vi "querey source settings menu.vi"(0 "Enable":bool=TRUE, 1 "subvi?":bool, 2 "Old Settings":T1, 5 "error in (no error)":errorcluster) -> (14 "Output cluster":T4={"Integer Timestamp"=0, "Einzel Voltage"=0.0, "Needle Voltage"=0.0, "Frequency"=1.0, "Width (ms) : 0.1 "=0.05, "Desired Amplitude (V)"=0.0, "X Voltage"=0.0, "Y Voltage"=0.0, "Settings ID"="", "ID#"=0} {"Needle Voltage" min=0.0 max=10.0 step=0.01 format="%.2g"; "Y Voltage" min=0.0 max=9.0 step=0.01 format="%.2g"; "X Voltage" min=0.0 max=9.0 step=0.01 format="%.2g"; "Einzel Voltage" min=0.0 max=10.0 step=0.01 format="%.2g"; "Desired Amplitude (V)" min=0.0 max=10.0 step=0.01 format="%5.2f"; "Width (ms) : 0.1" min=0.05 max=5.0 step=0.01 format="%6.2f"; "Frequency" min=1.0 max=100.0 step=0.01 format="%.1f"}, 15 "Cancel loading":bool caption="Cancel", 18 "OK":bool, 19 "error out":errorcluster)   [LabVIEW 2013]
doc: "Displays a standard dialog box that prompts users to enter information, such as a user name and password.\n--------------------\n\nThis Express VI is configured as follows:\n\nMessage to Display to the User:\nThe inputs are: \nNumber: Upper Timestamp Range\nNumber: Lower Timestamp Range\nNumber: Settings ID"
uses:
  Controls/dust_soruce_control.ctl
  <vilib>/Utility/miscctls.llb/LVPointTypeDef.ctl
  <vilib>/addons/database/Auxilliary.llb/DB Tools Cursor Type.ctl
  <vilib>/addons/database/Connection.llb/Conn Execute.vi
  <vilib>/addons/database/Recordset.llb/Rec Fetch Recordset Data (R).vi
  <vilib>/addons/database/Recordset.llb/Rec Destroy - Connection.vi
  <vilib>/addons/database/_DB Variant To Data/Database Variant To Data.xnode
  <vilib>/regexp/Match Regular Expression.xnode
  <vilib>/addons/database/NI_Database_API.lvlib
panel:
  out "Small Settings":cluster{"String":string, "Value":dbl}[](array[cluster])
  in  "Clear Filter":bool
  in  "Tag Filter":T2
  in  "Settings ID Type":T3(radio)
  in  "OK2":bool
  in  "Cancel":bool
  in  "Settings ID":i32(ring) items=["Any Settings ID."=-1, "Big Accelerator:  (time: 6/12/2014 3:08:20 PM; DT: Graphite-2-1)"=11, "Big Accelerator: test (time: 6/12/2014 11:46:17 AM;DT: Graphite-2-1)"=10, "Big Accelerator: test (time: 6/12/2014 10:56:33 AM;DT: Graphite-2-1)"=8, "Big Accelerator:  (time: 6/12/2014 10:56:28 AM;DT: Graphite-2-1)"=7, "Big Accelerator: olivine (saved at  1/29/2014 1:59:55 PM)"=6, "Big Accelerator: olivine (saved at  1/29/2014 1:53:03 PM)"=4, "Big Accelerator: test (saved at  1/29/2014 1:49:28 PM)"=2]
  in  "Lower Timestamp Range":timestamp
  in  "Upper Timestamp Range":timestamp
  out "Settings":cluster{"String":string, "Value":dbl}[](array[cluster])
  in  "Einzel Voltage":dbl
  in  "Needle Voltage":dbl
  in  "Frequency":dbl
  in  "Width (ms) : 0.1":dbl
  in  "Desired Amplitude (V)":dbl
  in  "X Voltage":dbl
  in  "Y Voltage":dbl
  out "Settings to be loaded":string
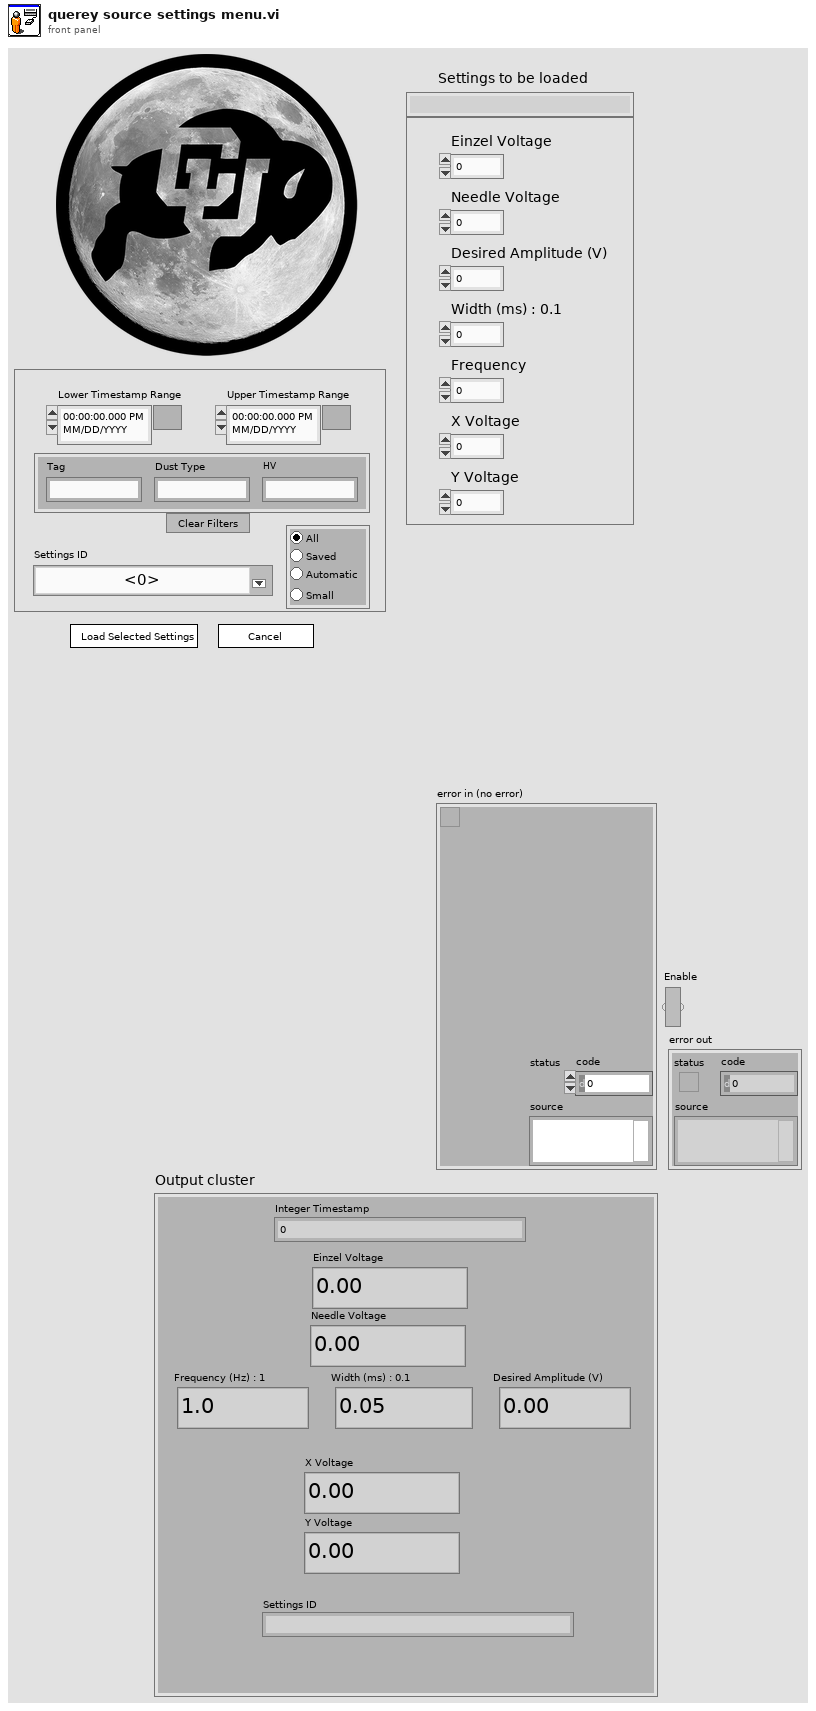
[diagram p1: front panel]
types:
  T1 = cluster{"Einzel":dbl, "X Voltage":dbl, "Y Voltage":dbl}
  T2 = cluster{"Tag":string, "Dust Type":string, "HV":string}
  T3 = enum32{"All", "Saved", "Automatic", "Small Accelerator"}
  T4 = typedef "dust_soruce_control.ctl" = cluster{"Integer Timestamp":u64, "Einzel Voltage":dbl, "Needle Voltage":dbl, "Frequency":dbl, "Width (ms) : 0.1 ":dbl, "Desired Amplitude (V)":dbl, "X Voltage":dbl, "Y Voltage":dbl, "Settings ID":string, "ID#":i32}
  T5 = typedef "LVPointTypeDef.ctl" = cluster{"Horizontal":i16, "Vertical":i16}
  T6 = enum32{"Invalid", "Standard", "Closed", "Hidden", "Minimized", "Maximized"}
  T7 = enum8{"Enabled", "Disabled", "Disabled and Grayed Out"}
  T8 = typedef "NI_Database_API.lvlib/DB Tools Cursor Type.ctl" = enum16{"forward-only", "keyset", "dynamic", "static"}
  T9 = typedef "NI_Database_API.lvlib/Conn ObjectReference.ctl" = refnum<k1>
  T10 = typedef "NI_Database_API.lvlib/Rec ObjectReference.ctl" = refnum<k1>
  T11 = typedef "dust_source_control_small.ctl" = cluster{"Integer Timestamp":u64, "Needle Voltage":dbl, "Frequency":dbl, "Width (ms) : 0.1 ":dbl, "Desired Amplitude (V)":dbl, "Settings ID":string, "ID#":i32}
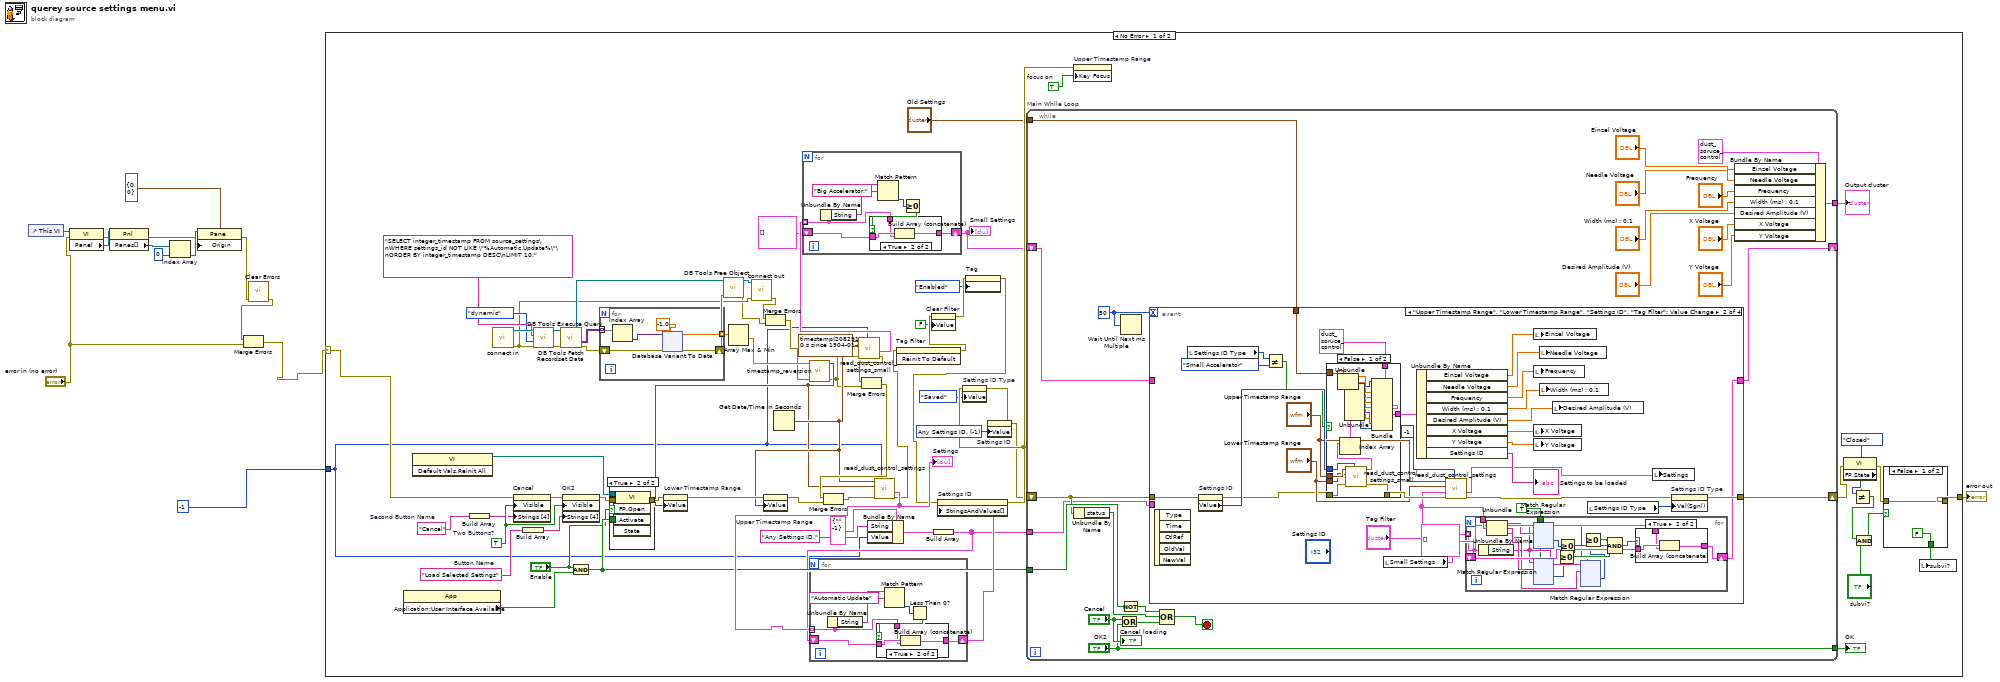
[diagram p0: block diagram]
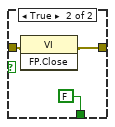
[diagram p4: hidden frame]
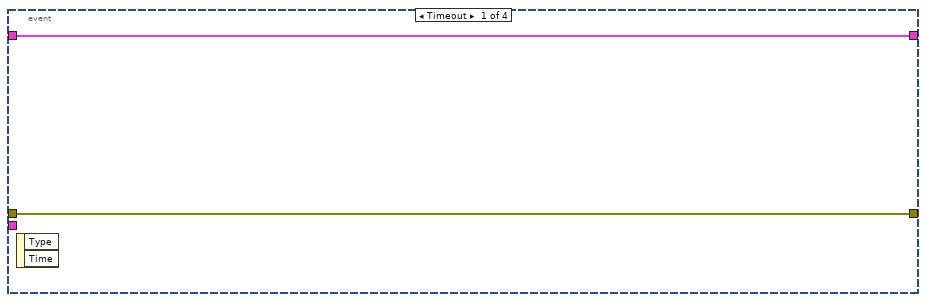
[diagram p6: hidden frame]
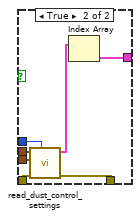
[diagram p7: hidden frame]
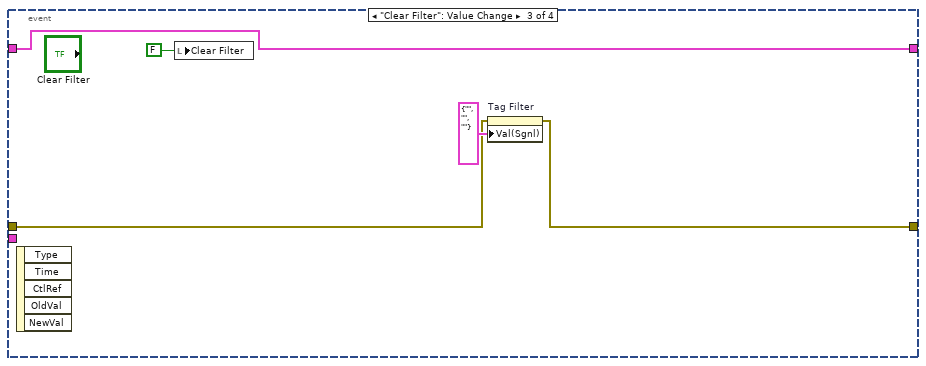
[diagram p9: hidden frame]
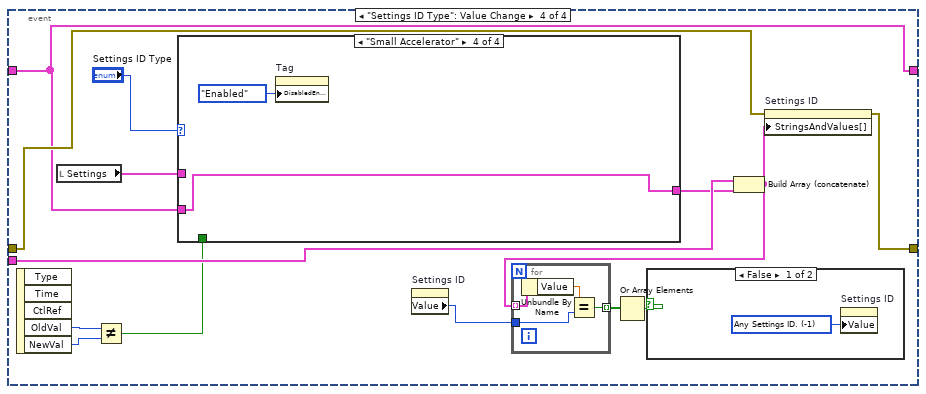
[diagram p10: hidden frame]
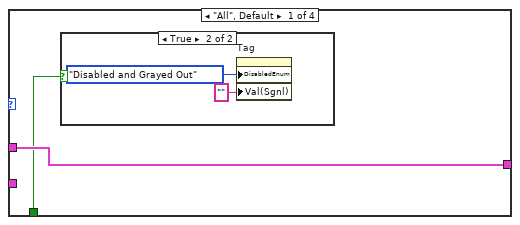
[diagram p12: hidden frame]
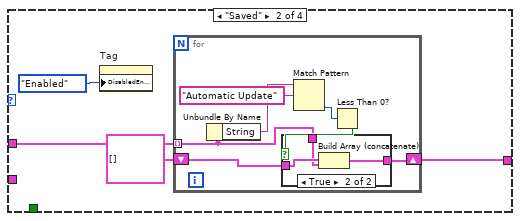
[diagram p14: hidden frame]
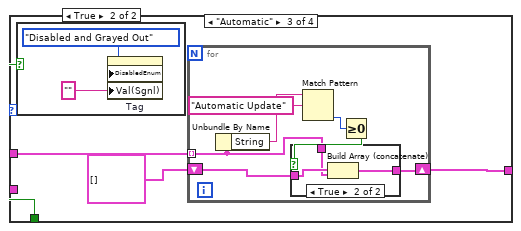
[diagram p16: hidden frame]
diagram:
  n1 = control-ref of="This VI"() -> (w4:refnum<vi>)
  n2 = property class="VI"(reference=w4, error in="error in (no error)") -> (error out=w5:errorcluster, "Panel"=w6:refnum<vi>)  [unwired: 1 out]
  n3 = property class="Pnl"(reference=w6, error in=w5) -> (error out=w7:errorcluster, "Panes[]"=w8:refnum<vi>[])  [unwired: 1 out]
  n4 = Index Array(array=w8, index=0) -> (element=w10:refnum<vi>)
  n5 = property class="Pane"(reference=w10, error in=w7, "Origin"=T5 {"Horizontal"=0, "Vertical"=0}) -> (error out=w12:errorcluster)  [unwired: 1 out]
  n6 = call <vilib>:"Clear Errors.vi"("error in (no error)"=w12) -> ("error out"=w1:errorcluster)  [unwired: 6 in]
  n7 = Merge Errors(w1, "error in (no error)") -> (w3:errorcluster)
  n8 = case shown="No Error" w3 {
    selector: w3 -> [w70 w663]
    tunnel: [w48 w663] -> w14
    tunnel: -1 ("Settings to be loaded") -> [w16 _]
    frame No Error {
      w43 = -1 items=["Any Settings ID."=-1, "Anna's Settings"=86, "Anna's Settings1"=87, "Test 'Test' \"Test\" test test."=97, "Test\""=91, "Test\""=92, "test 3"=82, "test 4"=83, "test mctesty"=88, "test mctesty"=89, "this is a \"test\" setting"=93] ("Settings ID")
      w78 = TRUE  # focus on
      w82 = "Cancel"  # Second Button Name
      w80 = "Load Selected Settings"  # Button Name
      w86 = TRUE  # Two Buttons?
      n9 = property class="App"() -> ("Application:User Interface Available"=w79:bool)  [unwired: 2 in, 2 out]
      n10 = invoke class="VI" method="Default Vals.Reinit All"() -> (reference out=w31:refnum<vi>)  [unwired: 3 in, 2 out]
      n11 = Build Array(w82) -> (w83:string[])
      n12 = call "connect in.vi"() -> ("error out"=w55:errorcluster, "Database Connection"=w65:T9)  [unwired: 7 in, 1 out]
      n13 = property on="Cancel" class="Bool"(error in=w70, "Visible"=w86, "Strings [4]"=w83) -> (error out=w84:errorcluster)  [unwired: 1 in, 1 out]
      n14 = Build Array(w80) -> (w81:string[])
      n15 = call-poly <vilib>:"DB Tools Execute Query.vi"("error in (no error)"=w55, "cursor type"=DB_Tools_Cursor_Type."dynamic", "SQL query"="SELECT integer_timestamp FROM source_settings\nWHERE settings_id NOT LIKE \"%Automatic Update%\"\nORDER BY integer_timestamp DESC\nLIMIT 10;" ("string"), "connection reference"=w65) -> ("error out"=w66:errorcluster, "recordset reference"=w67:T10)  [unwired: 4 in]
      n16 = call-poly <vilib>:"DB Tools Fetch Recordset Data.vi"("error in (no error)"=w66, "recordset reference"=w67) -> ("error out"=w61:errorcluster, "recordset data"=w62:variant[][], "recordset reference out"=w57:T10)  [unwired: 3 in]
      n17 = property on="OK2" class="Bool"(error in=w84, "Visible"=w86, "Strings [4]"=w81) -> (error out=w77:errorcluster)  [unwired: 1 in, 1 out]
      n18 = And(x="Enable", y=w79) -> (x .and. y?=w42:bool)
      n19 = for {
        tunnel: w62 -> [w123] mode=indexing
        tunnel: [w121] -> w60 mode=indexing
        shift-right: [w119] -> w56
        shift-left: w61 -> [w120]
        n20 = Index Array(array=w123) -> (element=w122:variant)  [unwired: 1 in]
        n21 = xnode "Database Variant To Data"("database variant"=w122, "error in (no error)"=w120, "type"=-1.0 ("Settings to be loaded")) -> ("data"=w121:dbl, "error out"=w119:errorcluster)
      }
      n22 = case shown="True" "Enable" {
        tunnel: w31 -> [_ w102]
        tunnel: w77 -> [w98 w101]
        tunnel: [w98 w100] -> w74
        tunnel: w42 -> [_ w99]
        frame False {
        }
        frame True {
          n23 = invoke class="VI" method="FP.Open"(reference=w102, error in=w101, "Activate"=w99) -> (error out=w100:errorcluster)  [unwired: 2 in, 4 out]
        }
      }
      n24 = call-poly <vilib>:"DB Tools Free Object.vi"("error in (no error)"=w56, "recordset reference"=w57) -> ("error out"=w54:errorcluster, "connection reference"=w58:T9)  [unwired: 8 in]
      n25 = Array Max & Min(array=w60) -> (min value=w59:dbl)  [unwired: 3 out]
      n26 = call "connect out.vi"("error in (no error)"=w55, "connection reference"=w58) -> ("error out"=w53:errorcluster)  [unwired: 9 in]
      n27 = Merge Errors(w53, w54) -> (w52:errorcluster)
      n28 = Get Date/Time In Seconds() -> (seconds since 1Jan1904=w25:timestamp)
      n29 = call "timestamp_reversion.vi"("error in (no error)"=w52, "Integer Timestamp"=w59) -> ("error out"=w23:errorcluster, "time stamp"=w24:timestamp)  [unwired: 7 in]
      n30 = property on="Lower Timestamp Range" class="AbsTime (strict)"(error in=w74, "Value"=w24) -> (error out=w75:errorcluster)  [unwired: 1 in, 1 out]
      n31 = property on="Upper Timestamp Range" class="AbsTime (strict)"(error in=w75, "Value"=w25) -> (error out=w51:errorcluster)  [unwired: 1 in, 1 out]
      n32 = call "read_dust_control_settings_small.vi"("Settings to be loaded"=w16, "error in (no error)"=w23, "Lower Timestamp Range"=timestamp(2082916800 s since 1904-01-01), "Upper Timestamp Range"=w25) -> ("error out"=w22:errorcluster, "Array"=w21:cluster{"String":string, "Value":dbl}[])  [unwired: 5 in, 1 out]
      n33 = for {
        tunnel: w21 -> [w89] mode=indexing
        shift-right: [w88] -> w18
        shift-left: cluster{"String":string, "Value":dbl}[] [] -> [w90]
        n34 = Unbundle By Name(w89) -> ("String"=w93:string)
        n35 = Match Pattern(string=w93, regular expression="Big Accelerator:") -> (offset past match=w87:i32)  [unwired: 1 in, 3 out]
        n36 = Greater Or Equal To 0?(x=w87) -> (x >= 0?=w91:bool)
        n37 = case shown="True" w91 {
          tunnel: w90 -> [w94 w97]
          tunnel: w89 -> [_ w96]
          tunnel: [w94 w95] -> w88
          frame False {
          }
          frame True {
            n38 = Build Array (concatenate)(w97, w96) -> (w95:cluster{"String":string, "Value":dbl}[])
          }
        }
      }
      "Small Settings" <- w18
      n39 = Merge Errors(w22, w23) -> (w50:errorcluster)
      n40 = Merge Errors(w50, w51) -> (w49:errorcluster)
      n41 = Bundle By Name(cluster=cluster{"String":string, "Value":i32} {"String"="", "Value"=-1}, "String"="Any Settings ID." ("Settings to be loaded"), "Value"=w16) -> (w71:cluster{"String":string, "Value":i32})
      n42 = call "read_dust_control_settings.vi"("Settings to be loaded"=w16, "error in (no error)"=w49, "Lower Timestamp Range"=w24, "Upper Timestamp Range"=w25) -> ("error out"=w39:errorcluster, "Array"=w46:cluster{"String":string, "Value":dbl}[])  [unwired: 5 in, 1 out]
      "Settings" <- w46
      n43 = invoke on="Tag Filter" class="Clust (strict)" method="Reinit To Default"(error in=w39) -> (error out=w38:errorcluster)  [unwired: 2 in, 2 out]
      n44 = property on="Clear Filter" class="Bool (strict)"(error in=w38, "Value"=FALSE ("Clear Filter")) -> (error out=w36:errorcluster)  [unwired: 1 in, 1 out]
      n45 = Build Array(w71) -> (w20:cluster{"String":string, "Value":i32}[])
      n46 = for {
        tunnel: w46 -> [w110] mode=indexing
        shift-right: [w109] -> w47
        shift-left: w20 -> [w111]
        n47 = Unbundle By Name(w110) -> ("String"=w114:string)
        n48 = Match Pattern(string=w114, regular expression="Automatic Update") -> (offset past match=w108:i32)  [unwired: 1 in, 3 out]
        n49 = Less Than 0?(x=w108) -> (x < 0?=w112:bool)
        n50 = case shown="True" w112 {
          tunnel: w111 -> [w115 w118]
          tunnel: w110 -> [_ w117]
          tunnel: [w115 w116] -> w109
          frame False {
          }
          frame True {
            n51 = Build Array (concatenate)(w118, w117) -> (w116:cluster{"String":string, "Value":dbl}[])
          }
        }
      }
      n52 = property on="Tag" class="Str"(error in=w36, "DisabledEnum"=T7."Enabled" ("Disabled")) -> (error out=w34:errorcluster)  [unwired: 1 in, 1 out]
      n53 = property on="Settings ID" class="Ring (strict)"(error in=w34, "StringsAndValues[]"=w47) -> (error out=w69:errorcluster)  [unwired: 1 in, 1 out]
      n54 = property on="Settings ID Type" class="RadioBtnsControl (strict)"(error in=w69, "Value"=enum32{"All", "Saved", "Automatic"}."Saved" ("Settings ID Type")) -> (error out=w45:errorcluster)  [unwired: 1 in, 1 out]
      n55 = property on="Settings ID" class="Ring (strict)"(error in=w45, "Value"=w43) -> (error out=w44:errorcluster)  [unwired: 1 in, 1 out]
      n56 = while "Main While Loop" {
        tunnel: ["OK2"] -> w85
        tunnel: w42 -> [w178]
        tunnel: w20 -> [w160]
        tunnel: [w169] -> w76
        shift-right: [w171] -> w30
        shift-left: w44 -> [w172]
        shift-right: [w158] -> _
        shift-left: w18 -> [w159]
        tunnel: "Old Settings" -> [w157]
        stop <- w176 stop-if-true
        w170 = u32 50 ("millisecond multiple")
        n57 = Unbundle By Name(w172) -> ("status"=w174:bool)
        n58 = Or(x="Cancel", y="OK2") -> (x .or. y?=w175:bool)
        n59 = Not(x=w178) -> (.not. x?=w177:bool)
        n60 = Wait Until Next ms Multiple(millisecond multiple=w170) -> ()  [unwired: 1 out]
        n61 = event shown="[1] \"Upper Timestamp Range\", \"Lower Timestamp Range\", \"Settings ID\", \"Tag Filter\": Value Change" {
          selector: _ -> [_ _ _ _]
          dyn-events: _ -> [_ _ _ _]
          timeout: w170 -> [_ _ _ _]
          tunnel: w172 -> [w181 w211 w603 w617]
          tunnel: [w181 w196 w602 w616] -> w171
          tunnel: w160 -> [_ _ _ w611]
          tunnel: w159 -> [w180 _ w601 w606]
          tunnel: [w180 w189 w601 w606] -> w158
          tunnel: w157 -> [_ w182 _ _]
          event Timeout {
            n62 = event-data() -> ()  [unwired: 1 in, 2 out]
          }
          event "Upper Timestamp Range", "Lower Timestamp Range", "Settings ID", "Tag Filter": Value Change {
            n63 = event-data() -> ()  [unwired: 1 in, 5 out]
            n64 = local read "Settings ID Type"() -> (w186:T3)
            n65 = property on="Settings ID" class="Ring (strict)"(error in=w211) -> (error out=w192:errorcluster, "Value"=w210:i32)  [unwired: 1 in, 1 out]
            n66 = Not Equal?(x=w186, y=T3."Small Accelerator") -> (x != y?=w184:bool)
            n67 = case shown="False" w184 {
              tunnel: w210 -> [w231 w237]
              tunnel: [w227 w236] -> w209
              tunnel: [w216 w235] -> w208
              tunnel: "Upper Timestamp Range" -> [w230 w234]
              tunnel: "Lower Timestamp Range" -> [w229 w233]
              tunnel: w192 -> [w228 w232]
              tunnel: T4 {"Integer Timestamp"=0, "Einzel Voltage"=0.0, "Needle Voltage"=0.0, "Frequency"=1.0, "Width (ms) : 0.1 "=0.05, "Desired Amplitude (V)"=0.0, "X Voltage"=0.0, "Y Voltage"=0.0, "Settings ID"="", "ID#"=0} ("Dust Source Controls") -> [w224 _]
              tunnel: w182 -> [w215 _]
              frame False {
                n68 = Unbundle(w215) -> ("Einzel"=w214:dbl, "X Voltage"=w213:dbl, "Y Voltage"=w212:dbl)
                n69 = call "read_dust_control_settings_small.vi"("Settings to be loaded"=w231, "error in (no error)"=w228, "Lower Timestamp Range"=w229, "Upper Timestamp Range"=w230) -> ("error out"=w227:errorcluster, "Dust Source Array"=w226:T11[])  [unwired: 5 in, 1 out]
                n70 = Index Array(array=w226) -> (element=w225:T11)  [unwired: 1 in]
                n71 = Unbundle(w225) -> ("Integer Timestamp"=w223:u64, "Needle Voltage"=w222:dbl, "Frequency"=w221:dbl, "Width (ms) : 0.1"=w220:dbl, "Desired Amplitude (V)"=w219:dbl, "Settings ID"=w218:string, "ID#"=w217:i32)
                n72 = Bundle(cluster=w224, "Integer Timestamp"=w223, "Einzel Voltage"=w214, "Needle Voltage"=w222, "Frequency"=w221, "Width (ms) : 0.1"=w220, "Desired Amplitude (V)"=w219, "X Voltage"=w213, "Y Voltage"=w212, "Settings ID"=w218, "ID#"=w217) -> (w216:T4)
              }
              frame True {
                n73 = call "read_dust_control_settings.vi"("Settings to be loaded"=w237, "error in (no error)"=w232, "Lower Timestamp Range"=w233, "Upper Timestamp Range"=w234) -> ("error out"=w236:errorcluster, "Dust Source Array"=w238:T4[])  [unwired: 5 in, 1 out]
                n74 = Index Array(array=w238) -> (element=w235:T4)  [unwired: 1 in]
              }
            }
            n75 = local read "Small Settings"() -> (w191:cluster{"String":string, "Value":dbl}[])
            n76 = Unbundle By Name(w208) -> ("Einzel Voltage"=w207:dbl, "Needle Voltage"=w206:dbl, "Frequency"=w205:dbl, "Width (ms) : 0.1"=w204:dbl, "Desired Amplitude (V)"=w203:dbl, "X Voltage"=w202:dbl, "Y Voltage"=w201:dbl, "Settings ID"=→"Settings to be loaded":string)
            n77 = call "read_dust_control_settings.vi"("Settings to be loaded"=-1, "error in (no error)"=w209, "Cluster"="Tag Filter", "Lower Timestamp Range"="Lower Timestamp Range", "Upper Timestamp Range"="Upper Timestamp Range") -> ("error out"=w197:errorcluster, "Array"=w195:cluster{"String":string, "Value":dbl}[])  [unwired: 4 in, 1 out]
            n78 = for {
              tunnel: w191 -> [w248] mode=indexing
              tunnel: "Tag Filter" -> [w254]
              shift-right: [w247] -> w189
              shift-left: cluster{"String":string, "Value":dbl}[] [] -> [w249]
              tunnel: TRUE -> [w240]
              n79 = Unbundle By Name(w248) -> ("String"=w242:string)
              n80 = Unbundle(w254) -> ("Tag"=w246:string, "Dust Type"=w244:string, "HV"=w243:string)
              n81 = xnode "Match Regular Expression"("input string"=w242, "regular expression"=w246, "ignore case? (F)"=w240) -> ("offset past match"=w245:i32)  [unwired: 3 in, 4 out]
              n82 = xnode "Match Regular Expression"("input string"=w242, "regular expression"=w244, "ignore case? (F)"=w240) -> ("offset past match"=w239:i32)  [unwired: 3 in, 4 out]
              n83 = Greater Or Equal To 0?(x=w239) -> (x >= 0?=w251:bool)
              n84 = Greater Or Equal To 0?(x=w245) -> (x >= 0?=w252:bool)
              n85 = xnode "Match Regular Expression"("input string"=w242, "regular expression"=w243, "ignore case? (F)"=w240) -> ("offset past match"=w241:i32)  [unwired: 3 in, 4 out]
              n86 = Greater Or Equal To 0?(x=w241) -> (x >= 0?=w253:bool)
              n87 = Compound Arithmetic op=AND(w253, w252, w251) -> (w250:bool)
              n88 = case shown="True" w250 {
                tunnel: w249 -> [w597 w600]
                tunnel: w248 -> [_ w599]
                tunnel: [w597 w598] -> w247
                frame False {
                }
                frame True {
                  n89 = Build Array (concatenate)(w600, w599) -> (w598:cluster{"String":string, "Value":dbl}[])
                }
              }
            }
            n90 = local write "Einzel Voltage"(w207) -> ()
            n91 = local write "Frequency"(w205) -> ()
            n92 = local write "X Voltage"(w202) -> ()
            n93 = local write "Y Voltage"(w201) -> ()
            n94 = local write "Needle Voltage"(w206) -> ()
            n95 = local write "Width (ms) : 0.1"(w204) -> ()
            n96 = local write "Desired Amplitude (V)"(w203) -> ()
            n97 = local read "Settings ID Type"() -> (w198:T3)
            n98 = local write "Settings"(w195) -> ()
            n99 = property on="Settings ID Type" class="RadioBtnsControl (strict)"(error in=w197, "Val(Sgnl)"=w198) -> (error out=w196:errorcluster)  [unwired: 1 in, 1 out]
          }
          event "Clear Filter": Value Change {
            n100 = event-data() -> ()  [unwired: 1 in, 5 out]
            n101 = local write "Clear Filter"(FALSE ("Clear Filter")) -> ()
            n102 = property on="Tag Filter" class="Clust (strict)"(error in=w603, "Val(Sgnl)"=T2 {"Tag"="", "Dust Type"="", "HV"=""} ("Value (Signaling)")) -> (error out=w602:errorcluster)  [unwired: 1 in, 1 out]
          }
          event "Settings ID Type": Value Change {
            n103 = event-data() -> ("OldVal"=w609:T3, "NewVal"=w608:T3)  [unwired: 1 in, 3 out]
            n104 = local read "Settings"() -> (w618:cluster{"String":string, "Value":dbl}[])
            n105 = Not Equal?(x=w609, y=w608) -> (x != y?=w607:bool)
            n106 = case shown="\"Small Accelerator\"" "Settings ID Type" {
              tunnel: w618 -> [w626 w632 w647 _]
              tunnel: [w626 w630 w646 w662] -> w610
              tunnel: w607 -> [w625 _ w644 _]
              tunnel: w606 -> [_ _ _ w662]
              frame "All", Default {
                n107 = case shown="True" w625 {
                  frame False {
                  }
                  frame True {
                    n108 = property on="Tag" class="Str"("DisabledEnum"=T7."Disabled and Grayed Out" ("Disabled"), "Val(Sgnl)"="" ("Value")) -> ()  [unwired: 2 in, 2 out]
                  }
                }
              }
              frame "Saved" {
                n109 = property on="Tag" class="Str"("DisabledEnum"=T7."Enabled" ("Disabled")) -> ()  [unwired: 2 in, 2 out]
                n110 = for {
                  tunnel: w632 -> [w634] mode=indexing
                  shift-right: [w633] -> w630
                  shift-left: cluster{"String":string, "Value":i32}[] [] -> [w635]
                  n111 = Unbundle By Name(w634) -> ("String"=w639:string)
                  n112 = Match Pattern(string=w639, regular expression="Automatic Update") -> (offset past match=w637:i32)  [unwired: 1 in, 3 out]
                  n113 = Less Than 0?(x=w637) -> (x < 0?=w636:bool)
                  n114 = case shown="True" w636 {
                    tunnel: w635 -> [w640 w643]
                    tunnel: w634 -> [_ w642]
                    tunnel: [w640 w641] -> w633
                    frame False {
                    }
                    frame True {
                      n115 = Build Array (concatenate)(w643, w642) -> (w641:cluster{"String":string, "Value":dbl}[])
                    }
                  }
                }
              }
              frame "Automatic" {
                n116 = case shown="True" w644 {
                  frame False {
                  }
                  frame True {
                    n117 = property on="Tag" class="Str"("DisabledEnum"=T7."Disabled and Grayed Out" ("Disabled"), "Val(Sgnl)"="" ("Value")) -> ()  [unwired: 2 in, 2 out]
                  }
                }
                n118 = for {
                  tunnel: w647 -> [w651] mode=indexing
                  shift-right: [w650] -> w646
                  shift-left: cluster{"String":string, "Value":i32}[] [] -> [w652]
                  n119 = Unbundle By Name(w651) -> ("String"=w656:string)
                  n120 = Match Pattern(string=w656, regular expression="Automatic Update") -> (offset past match=w654:i32)  [unwired: 1 in, 3 out]
                  n121 = Greater Or Equal To 0?(x=w654) -> (x >= 0?=w653:bool)
                  n122 = case shown="True" w653 {
                    tunnel: w652 -> [w657 w660]
                    tunnel: w651 -> [_ w659]
                    tunnel: [w657 w658] -> w650
                    frame False {
                    }
                    frame True {
                      n123 = Build Array (concatenate)(w660, w659) -> (w658:cluster{"String":string, "Value":dbl}[])
                    }
                  }
                }
              }
              frame "Small Accelerator" {
                n124 = property on="Tag" class="Str"("DisabledEnum"=T7."Enabled" ("Disabled")) -> ()  [unwired: 2 in, 2 out]
              }
            }
            n125 = property on="Settings ID" class="Ring (strict)"() -> ("Value"=w615:i32)  [unwired: 2 in, 2 out]
            n126 = Build Array (concatenate)(w611, w610) -> (w612:cluster{"String":string, "Value":dbl}[])
            n127 = for {
              tunnel: w612 -> [w623] mode=indexing
              tunnel: w615 -> [w621]
              tunnel: [w620] -> w614 mode=indexing
              n128 = Unbundle By Name(w623) -> ("Value"=w622:dbl)
              n129 = Equal?(x=w622, y=w621) -> (x = y?=w620:bool)
            }
            n130 = Or Array Elements(Boolean array=w614) -> (logical OR=w613:bool)
            n131 = case shown="False" w613 {
              frame False {
                w624 = i16 -1 items=["Any Settings ID."=-1, "Anna's Settings"=86, "Anna's Settings1"=87, "Test 'Test' \"Test\" test test."=97, "Test\""=91, "Test\""=92, "test 3"=82, "test 4"=83, "test mctesty"=88, "test mctesty"=89, "this is a \"test\" setting"=93] ("Settings ID")
                n132 = property on="Settings ID" class="Ring (strict)"("Value"=w624) -> ()  [unwired: 2 in, 2 out]
              }
              frame True {
              }
            }
            n133 = property on="Settings ID" class="Ring (strict)"(error in=w617, "StringsAndValues[]"=w612) -> (error out=w616:errorcluster)  [unwired: 1 in, 1 out]
          }
        }
        n134 = Compound Arithmetic op=OR(w177, w174, w175) -> (w176:bool)
        n135 = Bundle By Name(cluster=T4 {"Integer Timestamp"=0, "Einzel Voltage"=0.0, "Needle Voltage"=0.0, "Frequency"=1.0, "Width (ms) : 0.1 "=0.05, "Desired Amplitude (V)"=0.0, "X Voltage"=0.0, "Y Voltage"=0.0, "Settings ID"="", "ID#"=0} ("Output cluster"), "Einzel Voltage"="Einzel Voltage", "Needle Voltage"="Needle Voltage", "Frequency"="Frequency", "Width (ms) : 0.1"="Width (ms) : 0.1", "Desired Amplitude (V)"="Desired Amplitude (V)", "X Voltage"="X Voltage", "Y Voltage"="Y Voltage") -> (w169:T4)
        "Cancel loading" <- "Cancel"
      }
      "OK" <- w85
      "Output cluster" <- w76
      n136 = property on="Upper Timestamp Range" class="AbsTime (strict)"(error in=w69, "Key Focus"=w78) -> ()  [unwired: 1 in, 2 out]
      n137 = property class="VI"(error in=w30) -> (error out=w29:errorcluster, "FP.State"=w28:T6)  [unwired: 1 in, 1 out]
      n138 = Not Equal?(x=w28, y=T6."Closed") -> (x != y?=w26:bool)
      n139 = And(x=w26, y="subvi?") -> (x .and. y?=w32:bool)
      n140 = case shown="False" w32 {
        tunnel: w29 -> [w104 w107]
        tunnel: [w104 w106] -> w48
        tunnel: [FALSE ("subvi?") FALSE ("subvi?")] -> w33
        frame False {
        }
        frame True {
          n141 = invoke class="VI" method="FP.Close"(error in=w107) -> (error out=w106:errorcluster)  [unwired: 2 in, 2 out]
        }
      }
      n142 = local write "subvi?"(w33) -> ()
    }
    frame Error {
    }
  }
  "error out" <- w14
